vi "AlliGator Compute CV Mean & SDV.vi"(8 "Error In":errorcluster, 9 "Iteration":i32, 11 "CV Array in":dbl[](array[numeric])) -> (0 "Error Out":errorcluster, 1 "CV SDV Array":dbl[](array[numeric]), 3 "Average CV Array":dbl[](array[numeric]))   [LabVIEW 2021, in "AlliGator Lifetime & Other Parameters.lvlib"]
uses:
  AlliGator Lifetime & Other Parameters.lvlib
  <vilib>/Utility/error.llb/Error Cluster From Error Code.vi
  <vilib>/ErrorRing/Error Ring.xnode
  <vilib>/Analysis/NI_AALBase.lvlib
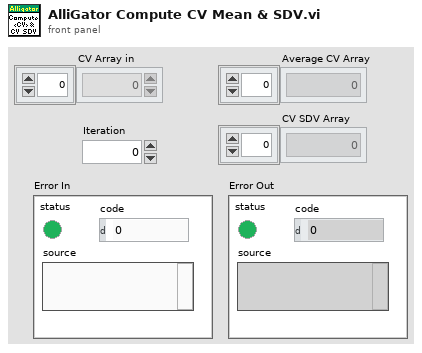
[diagram p1: front panel]
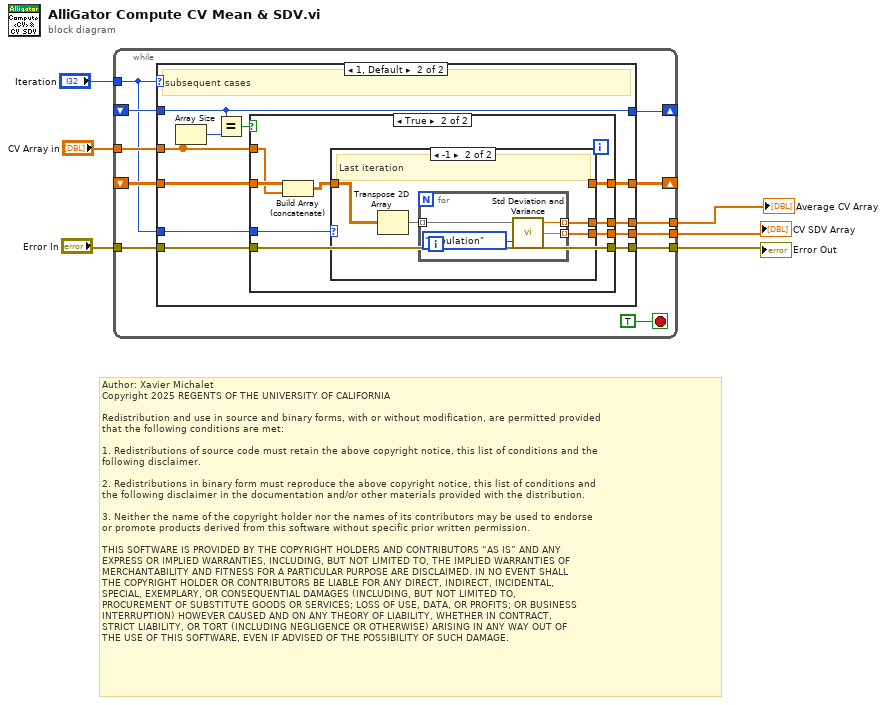
[diagram p0: block diagram]
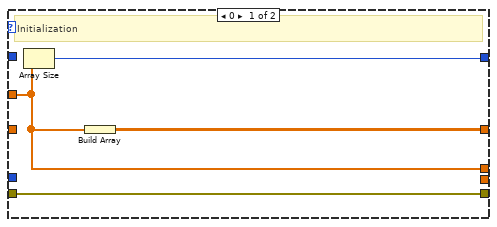
[diagram p2: hidden frame]
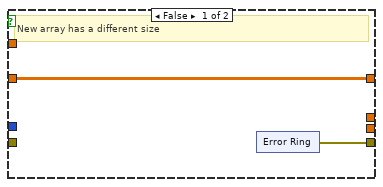
[diagram p3: hidden frame]
diagram:
  # "Author: Xavier Michalet\nCopyright 2025 REGENTS OF THE UNIVERSITY OF CALIFORNIA\n\nRedistribution and use in source and binary forms, with or without modification, are permitted provided\nthat the following conditions are met:\n\n1. Redistributions of source code must retain the above copyright notice, this list of conditions and the\nfollowing disclaimer.\n\n2. Redistributions in binary form must reproduce the above copyright notice, this list of conditions and\nthe following disclaimer in the documentation and/or other materials provided with the distribution.\n\n3. Neither the name of the copyright holder nor the names of its contributors may be used to endorse \nor promote products derived from this software without specific prior written permission.\n\nTHIS SOFTWARE IS PROVIDED BY THE COPYRIGHT HOLDERS AND CONTRIBUTORS “AS IS” AND ANY \nEXPRESS OR IMPLIED WARRANTIES, INCLUDING, BUT NOT LIMITED TO, THE IMPLIED WARRANTIES OF\nMERCHANTABILITY AND FITNESS FOR A PARTICULAR PURPOSE ARE DISCLAIMED. IN NO EVENT SHALL\nTHE COPYRIGHT HOLDER OR CONTRIBUTORS BE LIABLE FOR ANY DIRECT, INDIRECT, INCIDENTAL, \nSPECIAL, EXEMPLARY, OR CONSEQUENTIAL DAMAGES (INCLUDING, BUT NOT LIMITED TO, \nPROCUREMENT OF SUBSTITUTE GOODS OR SERVICES; LOSS OF USE, DATA, OR PROFITS; OR BUSINESS\nINTERRUPTION) HOWEVER CAUSED AND ON ANY THEORY OF LIABILITY, WHETHER IN CONTRACT, \nSTRICT LIABILITY, OR TORT (INCLUDING NEGLIGENCE OR OTHERWISE) ARISING IN ANY WAY OUT OF\nTHE USE OF THIS SOFTWARE, EVEN IF ADVISED OF THE POSSIBILITY OF SUCH DAMAGE."
  n1 = while {
    tunnel: "Iteration" -> [w7]
    shift-right: [w16] -> _
    shift-left: _ -> [w12]
    tunnel: "CV Array in" -> [w17]
    shift-right: [w15] -> _
    shift-left: _ -> [w14]
    tunnel: [w11] -> w4
    tunnel: "Error In" -> [w10]
    tunnel: [w9] -> w2
    tunnel: [w8] -> w1
    stop <- TRUE stop-if-true
    n2 = case shown="1, Default" w7 {
      tunnel: w17 -> [w18 w29]
      tunnel: [w21 w27] -> w16
      tunnel: [w20 w31] -> w15
      tunnel: w14 -> [_ w31]
      tunnel: w12 -> [_ w28]
      tunnel: [w19 w26] -> w11
      tunnel: w10 -> [w19 w25]
      tunnel: [w18 w24] -> w9
      tunnel: [_ w23] -> w8
      tunnel: w7 -> [_ w22]
      frame 0 {
        # "Initialization"
        n3 = Array Size(array=w18) -> (size(s)=w20:i32)
        n4 = Build Array(w18) -> (w21:dbl[][])
      }
      frame 1, Default {
        # "subsequent cases"
        n5 = Array Size(array=w29) -> (size(s)=w32:i32)
        n6 = Equal?(x=w31, y=w32) -> (x = y?=w30:bool)
        n7 = case shown="True" w30 {
          tunnel: w29 -> [_ w45]
          tunnel: w28 -> [w33 w46]
          tunnel: [w33 w39] -> w27
          tunnel: [w34 w44] -> w26
          tunnel: w25 -> [_ w44]
          tunnel: [_ w42] -> w24
          tunnel: [_ w41] -> w23
          tunnel: w22 -> [_ w40]
          frame False {
            # "New array has a different size"
            n8 = xnode "Error Ring"() -> ("error out"=w34:errorcluster)
          }
          frame True {
            n9 = Build Array (concatenate)(w46, w45) -> (w43:dbl[][])
            n10 = case shown="-1" w40 {
              tunnel: w43 -> [w47 w48]
              tunnel: [_ w50] -> w42
              tunnel: [_ w49] -> w41
              tunnel: [w47 _] -> w39
              frame 0, Default {
              }
              frame -1 {
                # "Last iteration"
                n11 = Transpose 2D Array(2D array=w48) -> (transposed array=w51:dbl[][])
                n12 = for {
                  tunnel: w51 -> [w55] mode=indexing
                  tunnel: [w53] -> w50 mode=indexing
                  tunnel: [w52] -> w49 mode=indexing
                  n13 = call <vilib>:"Std Deviation and Variance.vi"("X"=w55, "Weighting (Sample)"=enum16{"Sample", "Population"}."Population") -> ("mean"=w53:dbl, "standard deviation"=w52:dbl)  [unwired: 1 out]
                }
              }
            }
          }
        }
      }
    }
  }
  "Average CV Array" <- w2
  "CV SDV Array" <- w1
  "Error Out" <- w4
